vi "Gauge Sweep.vi"(8 "error in (no error)":errorcluster, 10 "Ctl Refnum":refnum<vi>) -> (0 "error out":errorcluster)   [LabVIEW 2011]
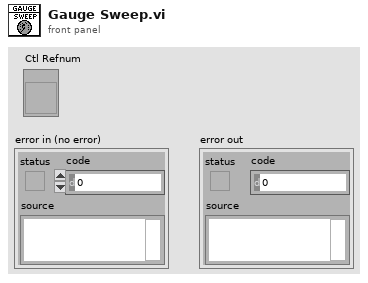
[diagram p1: front panel]
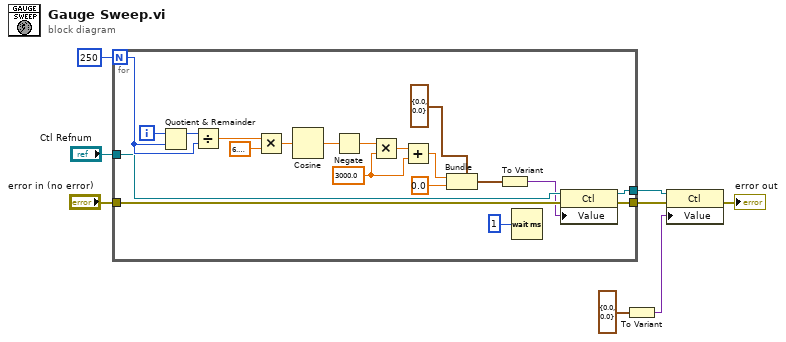
[diagram p0: block diagram]
diagram:
  n1 = for {
    N: 250 -> [w25]
    tunnel: "Ctl Refnum" -> [w17]
    tunnel: [w16] -> w5
    tunnel: [w15] -> w6
    tunnel: "error in (no error)" -> [w14]
    i -> [w27]
    w22 = 3000.0 ("y")
    n2 = Quotient & Remainder(x=w27, y=w25) -> (x-y*floor(x/y)=w26:i32)  [unwired: 1 out]
    n3 = Divide(x=w26, y=w25) -> (x/y=w24:dbl)
    n4 = Multiply(x=w24, y=6.283185307179586) -> (x*y=w20:dbl)
    n5 = Cosine(x=w20) -> (cos(x)=w19:dbl)
    n6 = Negate(x=w19) -> (-x=w18:dbl)
    n7 = Multiply(x=w18, y=w22) -> (x*y=w23:dbl)
    n8 = Add(x=w23, y=w22) -> (x+y=w10:dbl)
    n9 = Bundle(cluster=cluster{dbl, dbl} {0.0, 0.0} ("Shooter RPM"), w10, 0.0) -> (w11:cluster{dbl, dbl})
    n10 = To Variant(anything=w11) -> (Variant=w13:variant)
    n11 = Wait (ms)(milliseconds to wait=u32 1) -> ()  [unwired: 1 out]
    n12 = property class="Ctl"(reference=w17, error in=w14, "Value"=w13) -> (reference out=w16:refnum<vi>, error out=w15:errorcluster)
  }
  n13 = To Variant(anything=cluster{dbl, dbl} {0.0, 0.0} ("Shooter RPM")) -> (Variant=w2:variant)
  n14 = property class="Ctl"(reference=w5, error in=w6, "Value"=w2) -> (error out=→"error out":errorcluster)  [unwired: 1 out]
